vi "SaveCoarseGraph.vi"(10 "name or relative path":string, 11 "XYGraph in":refnum<vi>) -> ()   [LabVIEW 2013]
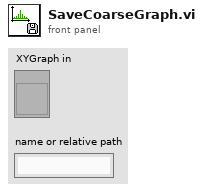
[diagram p1: front panel]
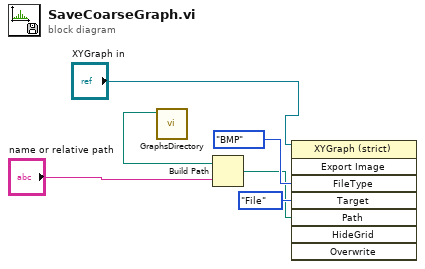
[diagram p0: block diagram]
diagram:
  n1 = call "GraphsDirectory.vi"() -> ("dup path"=w2:path)  [unwired: 11 in]
  n2 = Build Path(base path=w2, name or relative path="name or relative path") -> (appended path=w4:path)
  n3 = invoke on="Invoke Node" class="XYGraph (strict)" method="Export Image"(reference="XYGraph in", "FileType"=enum32{"BMP", "EPS", "EMF", "PICT"}."BMP" ("File Type"), "Target"=enum32{"File", "Clipboard"}."File", "Path"=w4) -> ()  [unwired: 4 in, 8 out]
